vi "Movement Checker.vi"(8 "error in":errorcluster) -> ()   [LabVIEW 2015]
uses:
  <vilib>/Rock Robotics/WPI/Utilities/WPI_GetSetVariantRefNum.vi
  Turret/Implementation/Turret Published Globals.vi
  Drive/Implementation/Drive Published Globals.vi
panel:
  in  "Maximum Speed in/sec":dbl=0.0003 format="%#_13g"
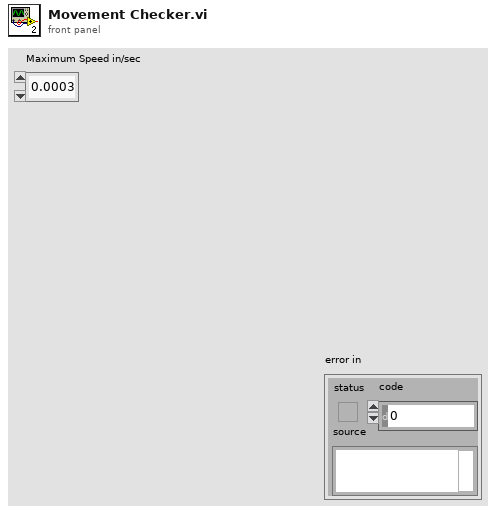
[diagram p1: front panel]
types:
  T1 = typedef "WPI_RobotDriveDevRef.ctl" = cluster{"DevStatus":errorcluster, "Motors[]":T2[], "Square Inputs":bool, "Max Output":dbl}
  T2 = typedef "WPI_MotorControlDeviceRef.ctl" = cluster{"DeviceStatus":errorcluster, "Type":T3, "PWM":cluster{"PWM Channel":T4, "DeadBand":T5}, "CAN":cluster{"Device Number":u8, "Control Mode":T6, "Semaphore":T7, "Max Vout":dbl, "TalonSRX Control Mode":T8}, "Invert":bool}
  T3 = typedef "WPI_MotorControlType.ctl" = enum16{"PWM", "CAN", "CANTalonSRX"}
  T4 = typedef "FPGA_DIOPWMChannel.ctl" = enum8{"PWM 0", "PWM 1", "PWM 2", "PWM 3", "PWM 4", "PWM 5", "PWM 6", "PWM 7", "PWM 8", "PWM 9", "PWM MXP 0", "PWM MXP 1", "PWM MXP 2", "PWM MXP 3", "PWM MXP 4", "PWM MXP 5", "PWM MXP 6", "PWM MXP 7", "PWM MXP 8", "PWM MXP 9", "Invalid"}
  T5 = typedef "WPI_PWMDeadband.ctl" = cluster{"Name":string, "maxPositivePwm":i32, "minPositivePwm":i32, "centerPwm":i32, "maxNegativePwm":i32, "minNegativePwm":i32, "angularRange":u16}
  T6 = typedef "WPI_CANJaguar_ControlMode.ctl" = enum8{"Percent VBus", "Current", "Speed", "Position", "Voltage"}
  T7 = typedef "Semaphore RefNum" = refnum<k1>
  T8 = typedef "WPI_CANTalonSRX_APIControlMode.ctl" = enum8{"Percent VBus", "Speed", "Position", "Slave", "Unchanged / Invalid", "Voltage Compensation", "Current", "Motion Profile"}
  T9 = typedef "WPI_CANTalonSRX_GlobalStatus.ctl" = cluster{"Applied Throttle":dbl, "Module Enabled":bool, "CAN Error":errorcluster, "Closed Loop Error":dbl, "Forward Limit Switch Closed":bool, "Reverse Limit Switch Closed":bool, "Sensor Position":dbl, "Sensor Velocity":dbl, "Current":dbl, "Sticky Fault - Over Temp":bool, "Sticky Fault - Under Voltage":bool, "Sticky Fault - Forward Limit":bool, "Sticky Fault - Reverse Limit":bool, "Sticky Fault - Forward Soft Limit":bool, "Sticky Fault - Reverse Soft Limit":bool, "Brake is Enabled":bool, "Encoder Position":dbl, "Encoder Velocity":dbl, "Encoder Index Count":dbl, "Encoder A Pin State":bool, "Encoder B Pin State":bool, "Encoder Index Pin State":bool, "Analog In":dbl, "Analog In Velocity":dbl, "Temperature (C)":dbl, "Battery Voltage":dbl, "Control 5 Is Supported":bool, "Current Profile Slot Select":dbl, "Pos Div 8":bool, "Vel Div 4":bool, "Pulse Width Position":i32, "Pulse Width Velocity":i32, "Pulse Width Rise To Rise (us)":i32, "Pulse Width Rise To Fall (us)":i32, "Mot Prof Active Is Under Run":bool, "Mot Prof Active Has Under Run":bool, "Mot Prof Active Is Last":bool, "Mot Prof Active Velocity Only":bool, "Mot Prof Active Is Valid":bool, "Mot Prof Buffer Is Full":bool, "Mot Prof Active Profile Slot Select":i32, "Mot Prof NextID":i32, "Mot Prof Count":i32, "Mot Prof Active Velocity":dbl, "Mot Prof Active Position":dbl, "Mot Prof Output Enable":i32}
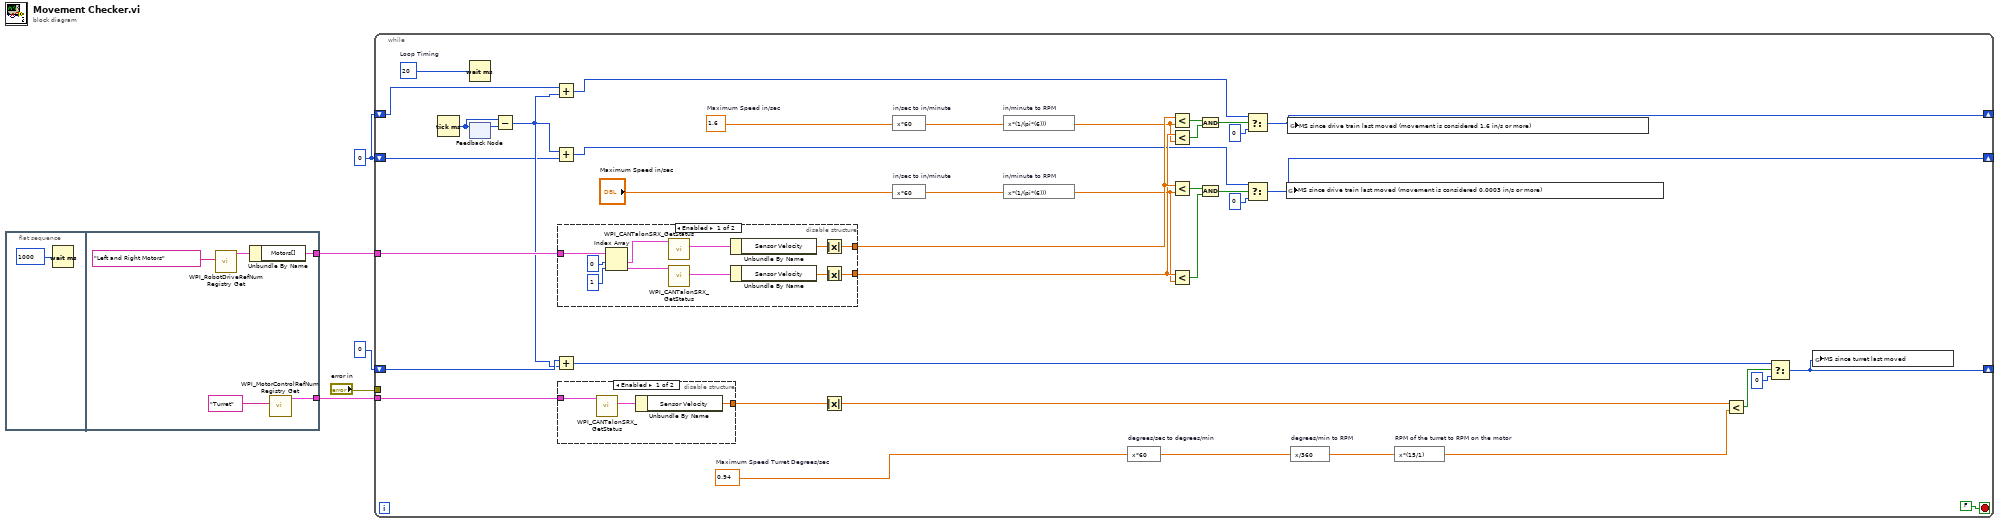
[diagram p0: block diagram]
diagram:
  w1 = 0
  n1 = flat-sequence {
    tunnel: [w10] -> w3
    tunnel: [w8] -> w2
    frame #0 {
      n2 = Wait (ms)(milliseconds to wait=1000) -> ()  [unwired: 1 out]
    }
    frame #1 {
      n3 = call <vilib>:"WPI_RobotDriveRefNum Registry Get.vi"("refnum name"="Left and Right Motors") -> ("RobotDriveDevRef"=w11:T1)  [unwired: 9 in, 1 out]
      n4 = Unbundle By Name(w11) -> ("Motors[]"=w10:T2[])
      n5 = call <vilib>:"WPI_MotorControlRefNum Registry Get.vi"("refnum name"="Turret") -> ("MotorControlDevRef"=w8:T2)  [unwired: 9 in, 1 out]
    }
  }
  n6 = while {
    shift-right: [w46] -> _
    shift-left: w1 -> [w51]
    shift-right: [w47] -> _
    shift-left: 0 -> [w50]
    tunnel: "error in" -> [_]
    tunnel: w3 -> [w45]
    tunnel: w2 -> [w44]
    shift-right: [w41] -> _
    shift-left: w1 -> [w42]
    stop <- FALSE stop-if-true
    w14 = 0.94  # Maximum Speed Turret Degrees/sec
    w24 = 1.6  # Maximum Speed in/sec
    w49 = 20  # Loop Timing
    n7 = Tick Count (ms)() -> (millisecond timer value=w40:u32)
    n8 = Wait (ms)(milliseconds to wait=w49) -> ()  [unwired: 1 out]
    n9 = feedback #1() -> (w39:u32)  [unwired: 1 in]
    n10 = feedback-in #1(w40) -> ()
    n11 = Subtract(x=w40, y=w39) -> (x-y=w43:u32)
    n12 = Add(x=w51, y=w43) -> (x+y=w34:u32)
    n13 = Add(x=w43, y=w42) -> (x+y=w28:u32)
    n14 = Add(x=w50, y=w43) -> (x+y=w15:u32)
    n15 = disable-structure shown="Enabled" {
      disable-tunnel: [w58 _] -> w30
      disable-tunnel: [w57 _] -> w29
      disable-tunnel: w45 -> [w55 _]
      frame Enabled {
        n16 = Index Array(array=w55, index #1=0 ("index"), index #2=1 ("index")) -> (element #1=w62:T2, element #2=w60:T2)
        n17 = call <vilib>:"WPI_CANTalonSRX_GetStatus.vi"("CAN Talon SRX Ref"=w62) -> ("Talon SRX Status"=w63:T9)  [unwired: 8 in, 2 out]
        n18 = call <vilib>:"WPI_CANTalonSRX_GetStatus.vi"("CAN Talon SRX Ref"=w60) -> ("Talon SRX Status"=w61:T9)  [unwired: 8 in, 2 out]
        n19 = Unbundle By Name(w63) -> ("Sensor Velocity"=w59:dbl)
        n20 = Unbundle By Name(w61) -> ("Sensor Velocity"=w56:dbl)
        n21 = Absolute Value(x=w59) -> (abs(x)=w58:dbl)
        n22 = Absolute Value(x=w56) -> (abs(x)=w57:dbl)
      }
      frame Disabled {
      }
    }
    n23 = disable-structure shown="Enabled" {
      disable-tunnel: [w53 _] -> w20
      disable-tunnel: w44 -> [w52 _]
      frame Enabled {
        n24 = call <vilib>:"WPI_CANTalonSRX_GetStatus.vi"("CAN Talon SRX Ref"=w52) -> ("Talon SRX Status"=w54:T9)  [unwired: 8 in, 2 out]
        n25 = Unbundle By Name(w54) -> ("Sensor Velocity"=w53:dbl)
      }
      frame Disabled {
      }
    }
    n26 = Absolute Value(x=w20) -> (abs(x)=w19:dbl)
    n27 = expression code="x*60" "in/sec to in/minute"(w24) -> (w21:dbl)
    n28 = expression code="x*60" "in/sec to in/minute"("Maximum Speed in/sec") -> (w22:dbl)
    n29 = expression code="x*(1/(pi*(6)))" "in/minute to RPM"(w21) -> (w23:dbl)
    n30 = expression code="x*(1/(pi*(6)))" "in/minute to RPM"(w22) -> (w26:dbl)
    n31 = expression code="x*60" "degrees/sec to degrees/min"(w14) -> (w12:dbl)
    n32 = Less?(x=w30, y=w23) -> (x < y?=w38:bool)
    n33 = Less?(x=w29, y=w23) -> (x < y?=w37:bool)
    n34 = Less?(x=w30, y=w26) -> (x < y?=w32:bool)
    n35 = Less?(x=w29, y=w26) -> (x < y?=w31:bool)
    n36 = And(x=w38, y=w37) -> (x .and. y?=w36:bool)
    n37 = And(x=w32, y=w31) -> (x .and. y?=w27:bool)
    n38 = Select(t=w34, s=w36, f=0) -> (s? t:f=w46:u32)
    n39 = Select(t=w28, s=w27, f=0) -> (s? t:f=w41:u32)
    n40 = global write "Drive Published Globals.vi" "MS since drive train last moved (movement is considered 0.0003 in/s or more)"(w41) -> ()
    n41 = global write "Drive Published Globals.vi" "MS since drive train last moved (movement is considered 1.6 in/s or more)"(w46) -> ()
    n42 = expression code="x/360" "degrees/min to RPM"(w12) -> (w13:dbl)
    n43 = expression code="x*(15/1)" "RPM of the turret to RPM on the motor"(w13) -> (w18:dbl)
    n44 = Less?(x=w19, y=w18) -> (x < y?=w17:bool)
    n45 = Select(t=w15, s=w17, f=0) -> (s? t:f=w47:u32)
    n46 = global write "Turret Published Globals.vi" "MS since turret last moved"(w47) -> ()
  }
